vi "setIntegrationTime.vi"(8 "error in (no error)":errorcluster, 11 "Electrometer in":refnum<class "Electrometer.lvclass">) -> (0 "error out":errorcluster, 3 "Electrometer out":refnum<class "Electrometer.lvclass">)   [LabVIEW 2016, in "Electrometer.lvclass"]
uses:
  Electrometer.lvclass
  ElectrometerConfiguration/ElectrometerInternalConfiguration.lvclass
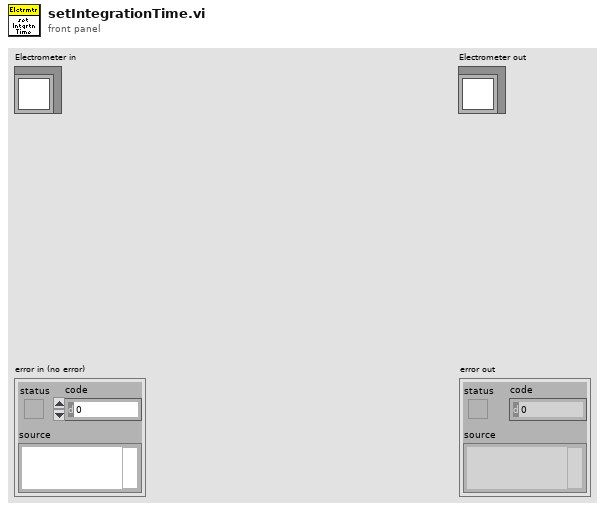
[diagram p1: front panel]
types:
  T1 = typedef "Electrometer.lvclass/Modes.ctl" = enum16{"Current", "Charge", "Voltage", "Resistance"}
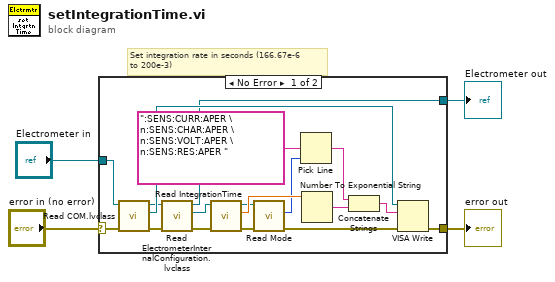
[diagram p0: block diagram]
diagram:
  # "Set integration rate in seconds (166.67e-6\nto 200e-3)"
  n1 = case shown="No Error" "error in (no error)" {
    selector: "error in (no error)" -> [w16 w24]
    tunnel: [w21 w24] -> w3
    tunnel: [w13 w23] -> w2
    tunnel: "Electrometer in" -> [w17 w23]
    frame No Error {
      n2 = call "Read COM.lvclass.vi"("error in (no error)"=w16, "Electrometer in"=w17) -> ("error out"=w10:errorcluster, "VISA"=w15:refnum<visa-resource-name>, "Electrometer out"=w14:refnum<class "Electrometer.lvclass">)  [unwired: 7 in]
      n3 = call-dynamic "Read ElectrometerInternalConfiguration.lvclass.vi"("error in (no error)"=w10, "Electrometer in"=w14) -> ("error out"=w11:errorcluster, "ElectrometerInternalConfiguration.lvclass"=w12:refnum<class "ElectrometerInternalConfiguration.lvclass">, "Electrometer out"=w13:refnum<class "Electrometer.lvclass">)  [unwired: 7 in]
      n4 = call-dynamic "Read IntegrationTime.vi"("error in (no error)"=w11, "ElectrometerInternalConfiguration in"=w12) -> ("error out"=w6:errorcluster, "IntegrationTime"=w9:dbl, "ElectrometerInternalConfiguration out"=w8:refnum<class "ElectrometerInternalConfiguration.lvclass">)  [unwired: 7 in]
      n5 = call-dynamic "Read Mode.vi"("error in (no error)"=w6, "ElectrometerInternalConfiguration in"=w8) -> ("error out"=w5:errorcluster, "Measurement Function (0: Current)"=w7:T1)  [unwired: 7 in, 1 out]
      n6 = Pick Line(multi-line string=":SENS:CURR:APER \n:SENS:CHAR:APER \n:SENS:VOLT:APER \n:SENS:RES:APER ", line index=w7) -> (output string=w20:string)  [unwired: 1 in]
      n7 = Number To Exponential String(number=w9) -> (E-format string=w19:string)  [unwired: 3 in]
      n8 = Concatenate Strings(w20, w19) -> (w18:string)
      n9 = VISA Write(VISA resource name=w15, write buffer=w18, error in (no error)=w5) -> (error out=w21:errorcluster)  [unwired: 2 out]
    }
    frame Error {
    }
  }
  "error out" <- w3
  "Electrometer out" <- w2
